vi "AOMStand_Analog.vi"(6 "stand Z vol backforth samp info":cluster{"Fs":dbl, "#s":dbl}={"Fs"=500000.0, "#s"=200000.0}, 8 "error in (no error)":errorcluster, 9 "AOM start blind percent (%)":dbl=70.0 min=10.0 max=90.0, 10 "AOM Blind percent (%)":dbl=0.1 min=0.1 max=100.0, 11 "Bi-Lateral Galvo xy scan frequency (Hz)":i16=500 min=500 max=500) -> (0 "error out":errorcluster)   [LabVIEW 2018]
panel:
  out "Preview":waveform(dbl)(graph)
  out "AOM Stand":waveform(dbl)
  out "AOM stand. value size":i32=400000
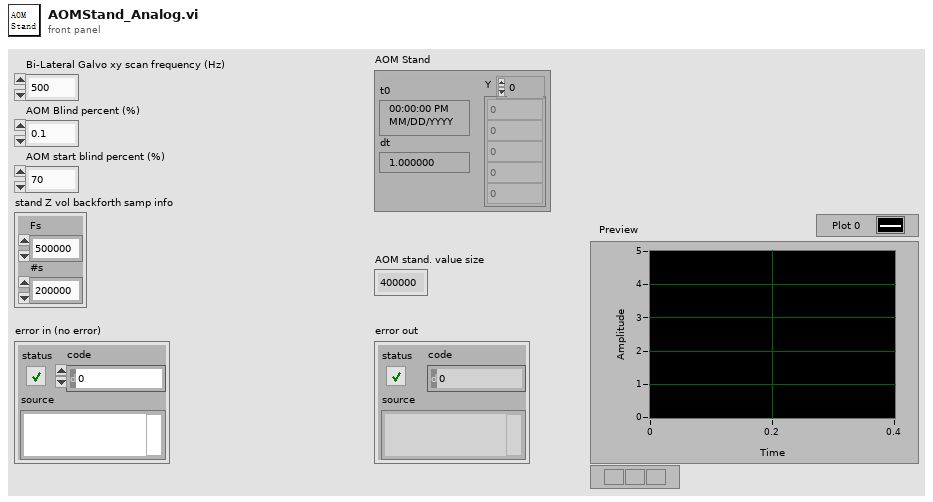
[diagram p1: front panel]
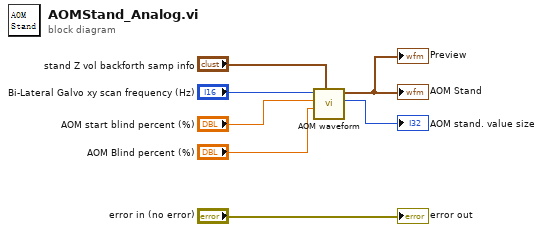
[diagram p0: block diagram]
diagram:
  n1 = call "AOM waveform.vi"("z stack 往复采样信息"="stand Z vol backforth samp info", "AOM Blind percent (%)"="AOM Blind percent (%)", "AOM start blind percent (%)"="AOM start blind percent (%)", "Bi-Lateral Galvo xy scan frequency (Hz)"="Bi-Lateral Galvo xy scan frequency (Hz)") -> ("数值"=→"AOM stand. value size":i32, "Waveform"=→"AOM Stand" →"Preview":waveform(dbl))  [unwired: 6 in]
  "error out" <- "error in (no error)"
